vi "Reference FPGA X410 loopback.vi"() -> ()   [LabVIEW 2023]
doc: "this VI is the top level of the FPGA.\n\nsubVIs placed at this level:\nmust have fixed-sized arrays.\ncontaining a class input (control) must NOT be left unconnected.\n\nconditional symbols supported for ease-of-use in building variations of the image are documented in a comment section and should be kept up-to-date."
uses:
  <vilib>/Platform/TimedLoop/XDataNode/timing_clust.ctl
  <vilib>/Platform/TimedLoop/XDataNode/nitl_modes.ctl
  <vilib>/Platform/TimedLoop/XDataNode/wakeup.ctl
  <instrlib>/_niInstr/DSP/v1/Shared/Public/IQ Data.ctl
  <vilib>/rvi/Emulation/niFpgaSctlEmulationGetInTimedLoop.vi
  <vilib>/rvi/Emulation/niFpgaEmulationReportErrorSimple.vi
  <vilib>/rvi/Emulation/niFpgaGetClockAttributes.vi
  <vilib>/rvi/Emulation/niFpgaCriticalErrorInLSC.vi
  <vilib>/Platform/TimedLoop/XDataNode/XDataNode.xnode
  <instrlib>/niUSRP/Reference FPGA/Instruction Framework/niUSRP Reference FPGA v1.lvclass
  <instrlib>/niUSRP/Reference FPGA/Rx DSP/niUSRP Rx DSP v2 FPGA.lvclass
  <instrlib>/niUSRP/Reference FPGA/Sync/niUSRP Rx Core v1 FPGA/niUSRP Sync v1 FPGA.lvclass
  <instrlib>/niUSRP/Reference FPGA/Tx DSP/niUSRP Tx DSP v2 FPGA.lvclass
  <vilib>/Platform/TimedLoop/XDataNode/XDNodeRunTimeDep.lvlib
  <instrlib>/niUSRP/Reference FPGA/Rx Core/niUSRP Rx Core v1 FPGA.lvclass
  <instrlib>/niUSRP/Reference FPGA/Stream Control/niUSRP Stream Control (DMA) v1 FPGA.lvclass
  <instrlib>/_niInstr/FIFO Register Bus/v1/FPGA/niInstr FIFO Register Bus v1 FPGA.lvclass
  <instrlib>/_niInstr/Instruction Framework/v1/FPGA/Collection Builder/Collection Builder.lvclass
  <instrlib>/niUSRP/Reference FPGA/Tx Core/niUSRP Tx Core v1 FPGA.lvclass
  <instrlib>/_niInstr/DSP/v1/Shared/niInstr DSP v1 Shared.lvlib
panel:
  out "fifo reg bus data 0":u64
  out "fifo reg bus status 0":u32
  in  "fifo reg bus ctrl 0":u32
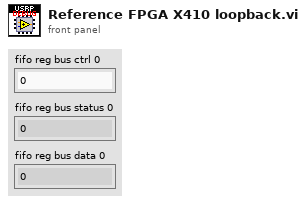
[diagram p1: front panel]
types:
  T1 = typedef "XDNodeRunTimeDep.lvlib/timing_clust.ctl" = cluster{"Expected End [f-1]":u64, "Actual End [f-1]":u64, "Finished Late? [f-1]":bool, "Expected End [i-1]":u64, "Actual End [i-1]":u64, "Finished Late? [i-1]":bool, "Expected Start [i]":u64, "Actual Start [i]":u64, "Expected Start [f]":u64, "Actual Start [f]":u64, "Source Name":string, "Structure Name":string, "Period":i64, "Deadline":i64, "Offset":i64, "Start":i64, "Priority":i32, "Timeout":i32, "Mode":T2, "Wakeup Reason":T3, "Error":errorcluster, "Source Type":string, "Secondary Source Type":string, "Global End Time":u64, "Global Start Time":u64, "Frame Duration":u64, "Iteration Duration":u64, "Assigned CPU":i32, "I/O Scan Engine Mode":u32}
  T2 = typedef "XDNodeRunTimeDep.lvlib/nitl_modes.ctl" = enum32{"No Change", "Process missed periods, maintain original phase", "Discard missed periods, maintain original phase", "Process missed periods, ignore original phase", "Discard missed periods, ignore original phase"}
  T3 = typedef "XDNodeRunTimeDep.lvlib/wakeup.ctl" = enum32{"Normal", "Aborted", "Asynchronous wakeup", "Timing source error", "Timed loop error", "Timeout"}
  T4 = typedef "niInstr DSP v1 Shared.lvlib/IQ Data.ctl" = cluster{"I":fxp<+/-,18,1>, "Q":fxp<+/-,18,1>, "overflow":bool}
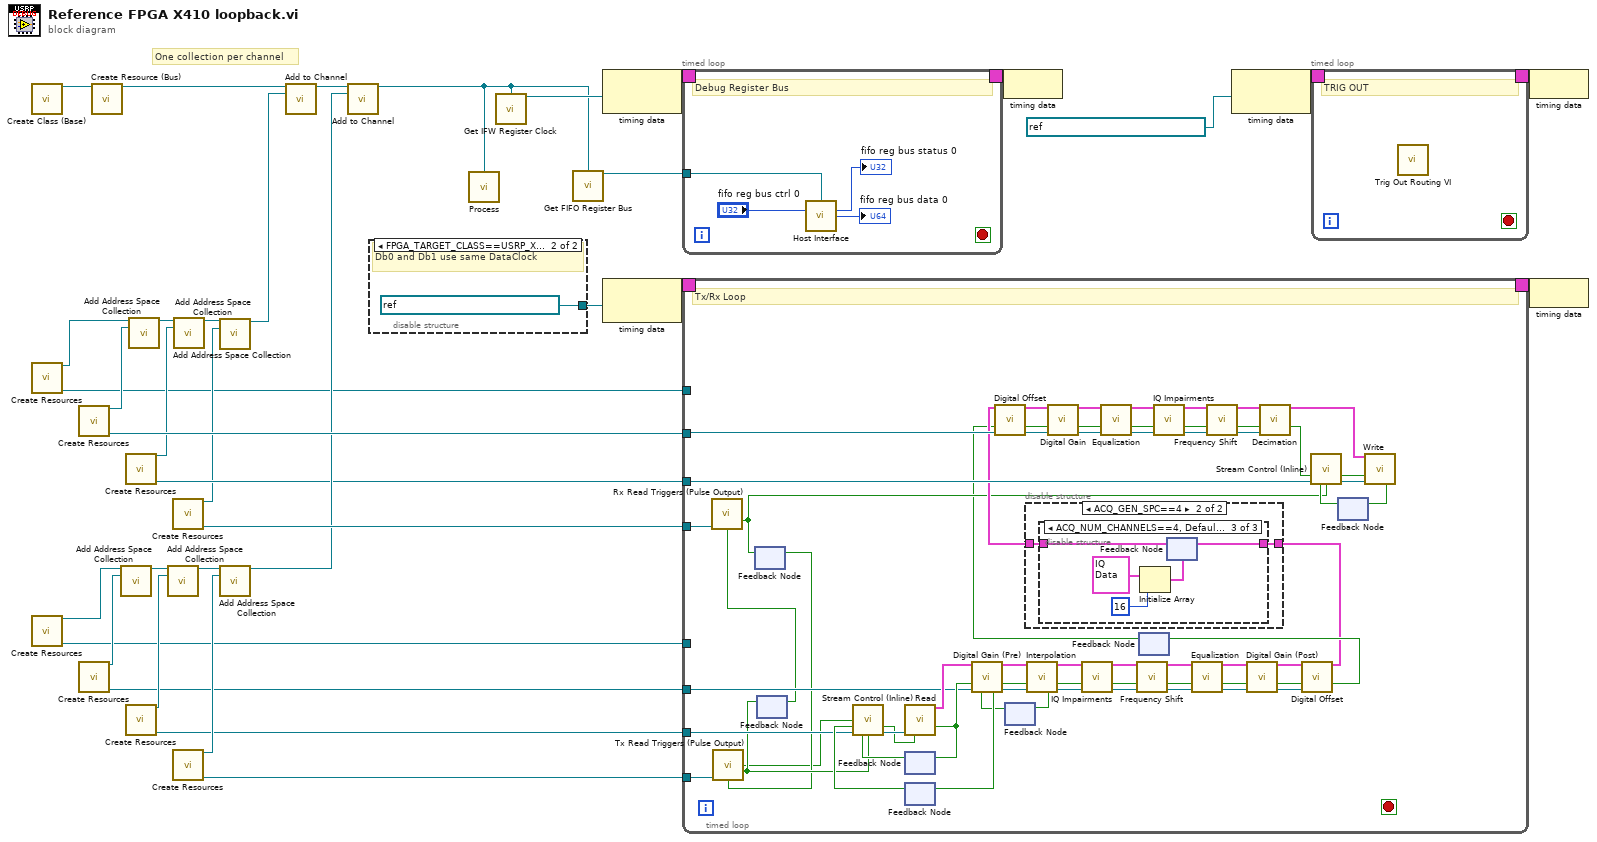
[diagram p0: block diagram]
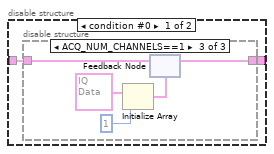
[diagram p2: hidden frame]
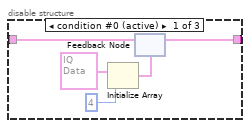
[diagram p3: hidden frame]
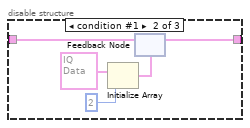
[diagram p4: hidden frame]
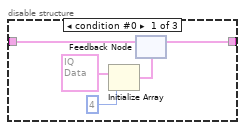
[diagram p5: hidden frame]
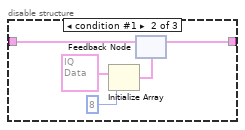
[diagram p6: hidden frame]
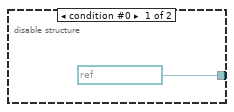
[diagram p7: hidden frame]
diagram:
  # "One collection per channel"
  n1 = call <instrlib>:"Create Class (Base).vi"() -> ("reference fpga"=w34:refnum<class "niUSRP Reference FPGA v1.lvclass">)  [unwired: 15 in]
  n2 = call <instrlib>:"Create Resources.vi"() -> ("channel collection builder"=w26:refnum<class "Collection Builder.lvclass">, "niVST Common Reference FPGA.lvclass"=w10:refnum<class "niUSRP Rx Core v1 FPGA.lvclass">)  [unwired: 14 in]
  n3 = call <instrlib>:"Create Resources.vi"() -> ("channel collection builder"=w17:refnum<class "Collection Builder.lvclass">, "niUSRP Tx Core"=w8:refnum<class "niUSRP Tx Core v1 FPGA.lvclass">)  [unwired: 14 in]
  n4 = call <instrlib>:"Create Resources.vi"() -> ("address space collection"=w30:refnum<class "Address Space Collection.lvclass">, "acq dsp session"=w31:refnum<class "niUSRP Rx DSP v2 FPGA.lvclass">)  [unwired: 14 in]
  n5 = call <instrlib>:"Create Resources.vi"() -> ("address space collection"=w16:refnum<class "Address Space Collection.lvclass">, "tx dsp"=w7:refnum<class "niUSRP Tx DSP v2 FPGA.lvclass">)  [unwired: 14 in]
  n6 = call-dynamic "Create Resource (Bus).vi"("reference fpga in"=w34) -> ("reference fpga out"=w29:refnum<class "niUSRP Reference FPGA v1.lvclass">)  [unwired: 14 in]
  n7 = call <instrlib>:"Add Address Space Collection.vi"("collection builder in"=w17, "address space collection"=w16) -> ("collection builder out"=w15:refnum<class "Collection Builder.lvclass">)  [unwired: 13 in]
  n8 = call <instrlib>:"Create Resources.vi"() -> ("address space collection"=w12:refnum<class "Address Space Collection.lvclass">, "stream session"=w20:refnum<class "niUSRP Stream Control (DMA) v1 FPGA.lvclass">)  [unwired: 14 in]
  n9 = call <instrlib>:"Create Resources.vi"() -> ("address space collection"=w19:refnum<class "Address Space Collection.lvclass">, "stream session"=w6:refnum<class "niUSRP Stream Control (DMA) v1 FPGA.lvclass">)  [unwired: 14 in]
  n10 = call <instrlib>:"Add Address Space Collection.vi"("collection builder in"=w26, "address space collection"=w30) -> ("collection builder out"=w28:refnum<class "Collection Builder.lvclass">)  [unwired: 13 in]
  n11 = call <instrlib>:"Add Address Space Collection.vi"("collection builder in"=w15, "address space collection"=w19) -> ("collection builder out"=w22:refnum<class "Collection Builder.lvclass">)  [unwired: 13 in]
  n12 = call <instrlib>:"Create Resources.vi"() -> ("address space collection"=w11:refnum<class "Address Space Collection.lvclass">, "stream control session"=w27:refnum<class "niUSRP Sync v1 FPGA.lvclass">)  [unwired: 14 in]
  n13 = call <instrlib>:"Create Resources.vi"() -> ("address space collection"=w18:refnum<class "Address Space Collection.lvclass">, "stream control session"=w5:refnum<class "niUSRP Sync v1 FPGA.lvclass">)  [unwired: 14 in]
  n14 = call <instrlib>:"Add Address Space Collection.vi"("collection builder in"=w28, "address space collection"=w12) -> ("collection builder out"=w25:refnum<class "Collection Builder.lvclass">)  [unwired: 13 in]
  n15 = call <instrlib>:"Add Address Space Collection.vi"("collection builder in"=w25, "address space collection"=w11) -> ("collection builder out"=w24:refnum<class "Collection Builder.lvclass">)  [unwired: 13 in]
  n16 = call <instrlib>:"Add Address Space Collection.vi"("collection builder in"=w22, "address space collection"=w18) -> ("collection builder out"=w21:refnum<class "Collection Builder.lvclass">)  [unwired: 13 in]
  n17 = call-dynamic "Add to Channel.vi"("reference fpga in"=w29, "collection builder in"=w24) -> ("reference fpga out"=w23:refnum<class "niUSRP Reference FPGA v1.lvclass">)  [unwired: 13 in]
  n18 = call-dynamic "Add to Channel.vi"("reference fpga in"=w23, "collection builder in"=w21) -> ("reference fpga out"=w9:refnum<class "niUSRP Reference FPGA v1.lvclass">)  [unwired: 13 in]
  n19 = disable-structure shown="FPGA_TARGET_CLASS==USRP_X410||FPGA_TARGET_CLASS==USRP_X410__EMBEDDED____UNSUPPORTED" {
    disable-tunnel: [refnum<k21> "Data Clock" ("Source Name") refnum<k21> "Daughterboard 0\\Data Clock" ("Source Name")] -> w2
    frame condition #0 {
    }
    frame condition #1 (active) {
      # "Db0 and Db1 use same DataClock"
    }
  }
  n20 = call <instrlib>:"Process.vi"("reference fpga"=w9) -> ()  [unwired: 15 in]
  n21 = call-dynamic "Get IFW Register Clock.vi"("reference fpga"=w9) -> ("ifw register clock"=w32:refnum<k21>)  [unwired: 14 in]
  n22 = call-dynamic "Get FIFO Register Bus.vi"("reference fpga"=w9) -> ("fifo register bus"=w33:refnum<class "niInstr FIFO Register Bus v1 FPGA.lvclass">)  [unwired: 14 in]
  n23 = node-c288 ("Input Node")(w32) -> (w36:T1)
  n24 = node-c288(w2) -> (w14:T1)
  n25 = timed-loop {
    timing: w36 -> [_]
    timing-out: [_] -> w35
    tunnel: w33 -> [w39]
    stop <- _ stop-if-true
    # "Debug Register Bus"
    n26 = call <instrlib>:"Host Interface.vi"("fifo register bus"=w39, "fifo reg bus ctrl 0"="fifo reg bus ctrl 0") -> ("fifo reg bus status 0"=→"fifo reg bus status 0":u32, "fifo reg bus data 0"=→"fifo reg bus data 0":u64)  [unwired: 12 in]
  }
  n27 = timed-loop "Acquisition Loop" {
    timing: w14 -> [_]
    timing-out: [_] -> w13
    tunnel: w31 -> [w98]
    tunnel: w10 -> [_]
    tunnel: w27 -> [w94]
    tunnel: w20 -> [w87]
    tunnel: w8 -> [_]
    tunnel: w7 -> [w61]
    tunnel: w6 -> [w60]
    tunnel: w5 -> [w59]
    stop <- _ stop-if-true
    # "Tx/Rx Loop"
    n28 = feedback #1() -> (w56:bool)  [unwired: 1 in]
    n29 = call-dynamic "Tx Read Triggers (Pulse Output).vi"("niUSRP Sync"=w59, "external trigger"=w56) -> ("future trigger"=w45:bool, "output valid"=w58:bool)  [unwired: 10 in, 2 out]
    n30 = feedback #2() -> (w57:bool)  [unwired: 1 in]
    n31 = call-dynamic "Rx Read Triggers (Pulse Output).vi"("niUSRP Sync"=w94, "external trigger"=w57) -> ("output valid"=w49:bool)  [unwired: 11 in, 2 out]
    n32 = feedback-in #1(w49) -> ()
    n33 = feedback-in #2(w58) -> ()
    n34 = feedback #3() -> (w62:bool)  [unwired: 1 in]
    n35 = feedback #4() -> (w63:bool)  [unwired: 1 in]
    n36 = call <instrlib>:"Stream Control (Inline).vi"("future trigger"=w45, "input valid"=w63, "stream control"=w60, "ready for output"=w62, "trigger"=w58) -> ("stream"=w65:bool, "stream control"=w72:refnum<class "niUSRP Stream Control (DMA) v1 FPGA.lvclass">)  [unwired: 7 in, 2 out]
    n37 = call <instrlib>:"Read.vi"("stream control"=w72, "ready for output"=w65) -> ("data out"=w74:T4[], "output valid"=w64:bool)  [unwired: 11 in, 1 out]
    n38 = feedback-in #3(w64) -> ()
    n39 = feedback #5() -> (w51:bool)  [unwired: 1 in]
    n40 = call-dynamic "Digital Gain (Pre).vi"("data in"=w74, "input valid"=w64, "gen in"=w61, "ready for output (T)"=w51) -> ("data out"=w53:T4[], "output valid"=w55:bool, "ready for input"=w73:bool, "gen out"=w54:refnum<class "niUSRP Tx DSP v2 FPGA.lvclass">)  [unwired: 8 in]
    n41 = feedback-in #4(w73) -> ()
    n42 = call-dynamic "Interpolation.vi"("data in"=w53, "input valid"=w55, "gen in"=w54) -> ("data out"=w83:T4[], "output valid"=w76:bool, "ready for input"=w52:bool, "gen out"=w75:refnum<class "niUSRP Tx DSP v2 FPGA.lvclass">)  [unwired: 9 in]
    n43 = feedback-in #5(w52) -> ()
    n44 = call-dynamic "IQ Impairments.vi"("data in"=w83, "input valid"=w76, "gen in"=w75) -> ("data out"=w71:T4[], "output valid"=w68:bool, "gen out"=w69:refnum<class "niUSRP Tx DSP v2 FPGA.lvclass">)  [unwired: 9 in, 1 out]
    n45 = call-dynamic "Frequency Shift.vi"("data in"=w71, "input valid"=w68, "gen in"=w69) -> ("data out"=w70:T4[], "output valid"=w67:bool, "gen out"=w66:refnum<class "niUSRP Tx DSP v2 FPGA.lvclass">)  [unwired: 9 in, 1 out]
    n46 = feedback #6() -> (w47:bool)  [unwired: 1 in]
    n47 = call-dynamic "Equalization.vi"("data in"=w70, "input valid"=w67, "gen in"=w66) -> ("data out"=w82:T4[], "output valid"=w77:bool, "gen out"=w78:refnum<class "niUSRP Tx DSP v2 FPGA.lvclass">)  [unwired: 9 in, 1 out]
    n48 = call-dynamic "Digital Gain (Post).vi"("data in"=w82, "input valid"=w77, "gen in"=w78) -> ("data out"=w81:T4[], "output valid"=w79:bool, "gen out"=w80:refnum<class "niUSRP Tx DSP v2 FPGA.lvclass">)  [unwired: 9 in, 1 out]
    n49 = call-dynamic "Digital Offset.vi"("data in"=w81, "input valid"=w79, "gen in"=w80) -> ("data out"=w46:T4[], "output valid"=w48:bool)  [unwired: 9 in, 2 out]
    n50 = disable-structure shown="ACQ_GEN_SPC==4" {
      disable-tunnel: [w109 w126] -> w50
      disable-tunnel: w46 -> [w108 w125]
      frame condition #0 {
        n51 = disable-structure shown="ACQ_NUM_CHANNELS==1" {
          disable-tunnel: [w114 w119 w124] -> w109
          disable-tunnel: w108 -> [w113 w118 w123]
          frame condition #0 (active) {
            n52 = Initialize Array(T4 {"I"=0.0, "Q"=0.0, "overflow"=FALSE} ("IQ data"), 4 ("dimension size")) -> (w110:T4[])
            n53 = feedback #7(w110) -> (w114:T4[])
            n54 = feedback-in #7(w113) -> ()
          }
          frame condition #1 {
            n55 = Initialize Array(T4 {"I"=0.0, "Q"=0.0, "overflow"=FALSE} ("IQ data"), 2 ("dimension size")) -> (w115:T4[])
            n56 = feedback #8(w115) -> (w119:T4[])
            n57 = feedback-in #8(w118) -> ()
          }
          frame condition #2 {
            n58 = Initialize Array(T4 {"I"=0.0, "Q"=0.0, "overflow"=FALSE} ("IQ data"), 1 ("dimension size")) -> (w120:T4[])
            n59 = feedback #9(w120) -> (w124:T4[])
            n60 = feedback-in #9(w123) -> ()
          }
        }
      }
      frame condition #1 (active) {
        n61 = disable-structure shown="ACQ_NUM_CHANNELS==4, Default" {
          disable-tunnel: [w131 w136 w141] -> w126
          disable-tunnel: w125 -> [w130 w135 w140]
          frame condition #0 {
            n62 = Initialize Array(T4 {"I"=0.0, "Q"=0.0, "overflow"=FALSE} ("IQ data"), 4 ("dimension size")) -> (w127:T4[])
            n63 = feedback #10(w127) -> (w131:T4[])
            n64 = feedback-in #10(w130) -> ()
          }
          frame condition #1 {
            n65 = Initialize Array(T4 {"I"=0.0, "Q"=0.0, "overflow"=FALSE} ("IQ data"), 8 ("dimension size")) -> (w132:T4[])
            n66 = feedback #11(w132) -> (w136:T4[])
            n67 = feedback-in #11(w135) -> ()
          }
          frame condition #2 (active) {
            n68 = Initialize Array(T4 {"I"=0.0, "Q"=0.0, "overflow"=FALSE} ("IQ data"), 16 ("dimension size")) -> (w137:T4[])
            n69 = feedback #12(w137) -> (w141:T4[])
            n70 = feedback-in #12(w140) -> ()
          }
        }
      }
    }
    n71 = call-dynamic "Digital Offset.vi"("data in"=w50, "input valid"=w47, "acq in"=w98) -> ("data out"=w107:T4[], "output valid"=w106:bool, "acq out"=w105:refnum<class "niUSRP Rx DSP v2 FPGA.lvclass">)  [unwired: 9 in, 1 out]
    n72 = call-dynamic "Digital Gain.vi"("data in"=w107, "input valid"=w106, "acq in"=w105) -> ("data out"=w102:T4[], "output valid"=w103:bool, "acq out"=w104:refnum<class "niUSRP Rx DSP v2 FPGA.lvclass">)  [unwired: 9 in, 1 out]
    n73 = call-dynamic "Equalization.vi"("data in"=w102, "input valid"=w103, "acq in"=w104) -> ("data out"=w101:T4[], "output valid"=w100:bool, "acq out"=w99:refnum<class "niUSRP Rx DSP v2 FPGA.lvclass">)  [unwired: 9 in, 1 out]
    n74 = feedback-in #6(w48) -> ()
    n75 = call-dynamic "IQ Impairments.vi"("data in"=w101, "input valid"=w100, "acq in"=w99) -> ("data out"=w93:T4[], "output valid"=w91:bool, "acq out"=w90:refnum<class "niUSRP Rx DSP v2 FPGA.lvclass">)  [unwired: 9 in, 1 out]
    n76 = call-dynamic "Frequency Shift.vi"("data in"=w93, "input valid"=w91, "acq in"=w90) -> ("data out"=w92:T4[], "output valid"=w88:bool, "acq out"=w89:refnum<class "niUSRP Rx DSP v2 FPGA.lvclass">)  [unwired: 9 in, 1 out]
    n77 = call-dynamic "Decimation.vi"("data in"=w92, "input valid"=w88, "acq in"=w89) -> ("data out"=w84:T4[], "output valid"=w95:bool)  [unwired: 9 in, 2 out]
    n78 = feedback #13() -> (w85:bool)  [unwired: 1 in]
    n79 = call <instrlib>:"Stream Control (Inline).vi"("input valid"=w95, "stream control"=w87, "ready for output"=w85, "trigger"=w49) -> ("stream"=w86:bool, "stream control"=w96:refnum<class "niUSRP Stream Control (DMA) v1 FPGA.lvclass">)  [unwired: 8 in, 2 out]
    n80 = call <instrlib>:"Write.vi"("data in"=w84, "input valid"=w86, "stream control"=w96) -> ("ready for input"=w97:bool)  [unwired: 11 in, 1 out]
    n81 = feedback-in #13(w97) -> ()
  }
  n82 = node-c288(w35) -> ()
  n83 = node-c288 ("Input Node")(refnum<k21> "Daughterboard 0\\Data Clock" ("Source Name")) -> (w4:T1)
  n84 = timed-loop {
    timing: w4 -> [_]
    timing-out: [_] -> w3
    stop <- _ stop-if-true
    # "TRIG OUT"
    n85 = call <instrlib>:"Trig Out Routing VI.vi"() -> ()  [unwired: 16 in]
  }
  n86 = node-c288(w3) -> ()
  n87 = node-c288(w13) -> ()
